vi "KeeperDefPosSkillVSS.vi"(8 "error in (no error)":errorcluster, 9 "Game":refnum<class "Game.lvclass">, 10 "Robot in":refnum<class "Robot.lvclass">, 11 "KeeperDefPosSkillVSS in":refnum<class "KeeperDefPosSkillVSS.lvclass">) -> (0 "error out":errorcluster, 2 "Robot out":refnum<class "Robot.lvclass">, 3 "KeeperDefPosSkillVSS out":refnum<class "KeeperDefPosSkillVSS.lvclass">)   [LabVIEW 2020, in "KeeperDefPosSkillVSS.lvclass"]
uses:
  KeeperDefPosSkillVSS.lvclass
  Robot_class/Robot.lvclass
  Game_class/Game.lvclass
  Utilities_class/Utilities.lvclass
  Game_class/Game.lvclass/Game.ctl
  Ball_class/Ball.lvclass/Ball.ctl
  Object_class/Object.lvclass/Object.ctl
  Robot_class/Robot.lvclass/Robot.ctl
  Game_class/Read FieldRef.vi
  Game_class/Read BallRef.vi
  Ball_class/Read v_x.vi
  Ball_class/Read v_y.vi
  Object_class/Read pos_est_y.vi
  Object_class/Read y.vi
  Object_class/Read x.vi
  Robot_class/Write dest_x.vi
  Robot_class/Write dest_y.vi
  Robot_class/Write dest_orientation.vi
  Ball_class/Ball.lvclass
  C:/Users/lucio/Desktop/Horie/ROBOIME/VSS_AI/Object_class/Object.lvclass
  Field_class/Field.lvclass
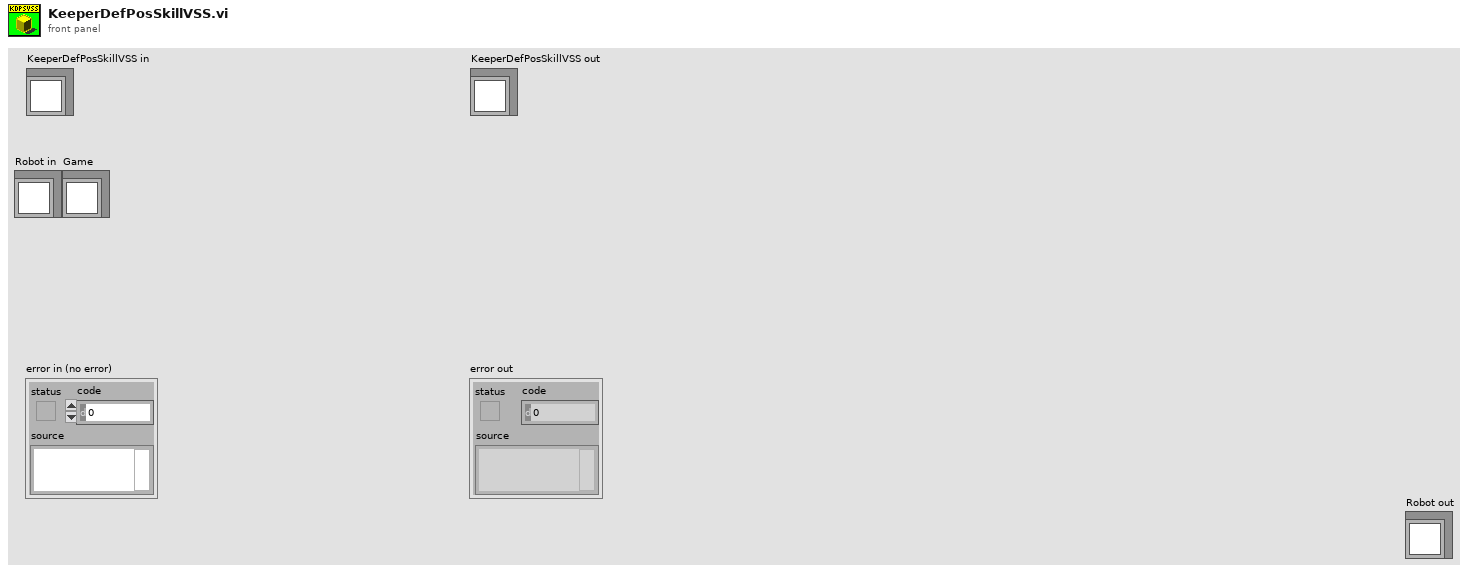
[diagram p1: front panel]
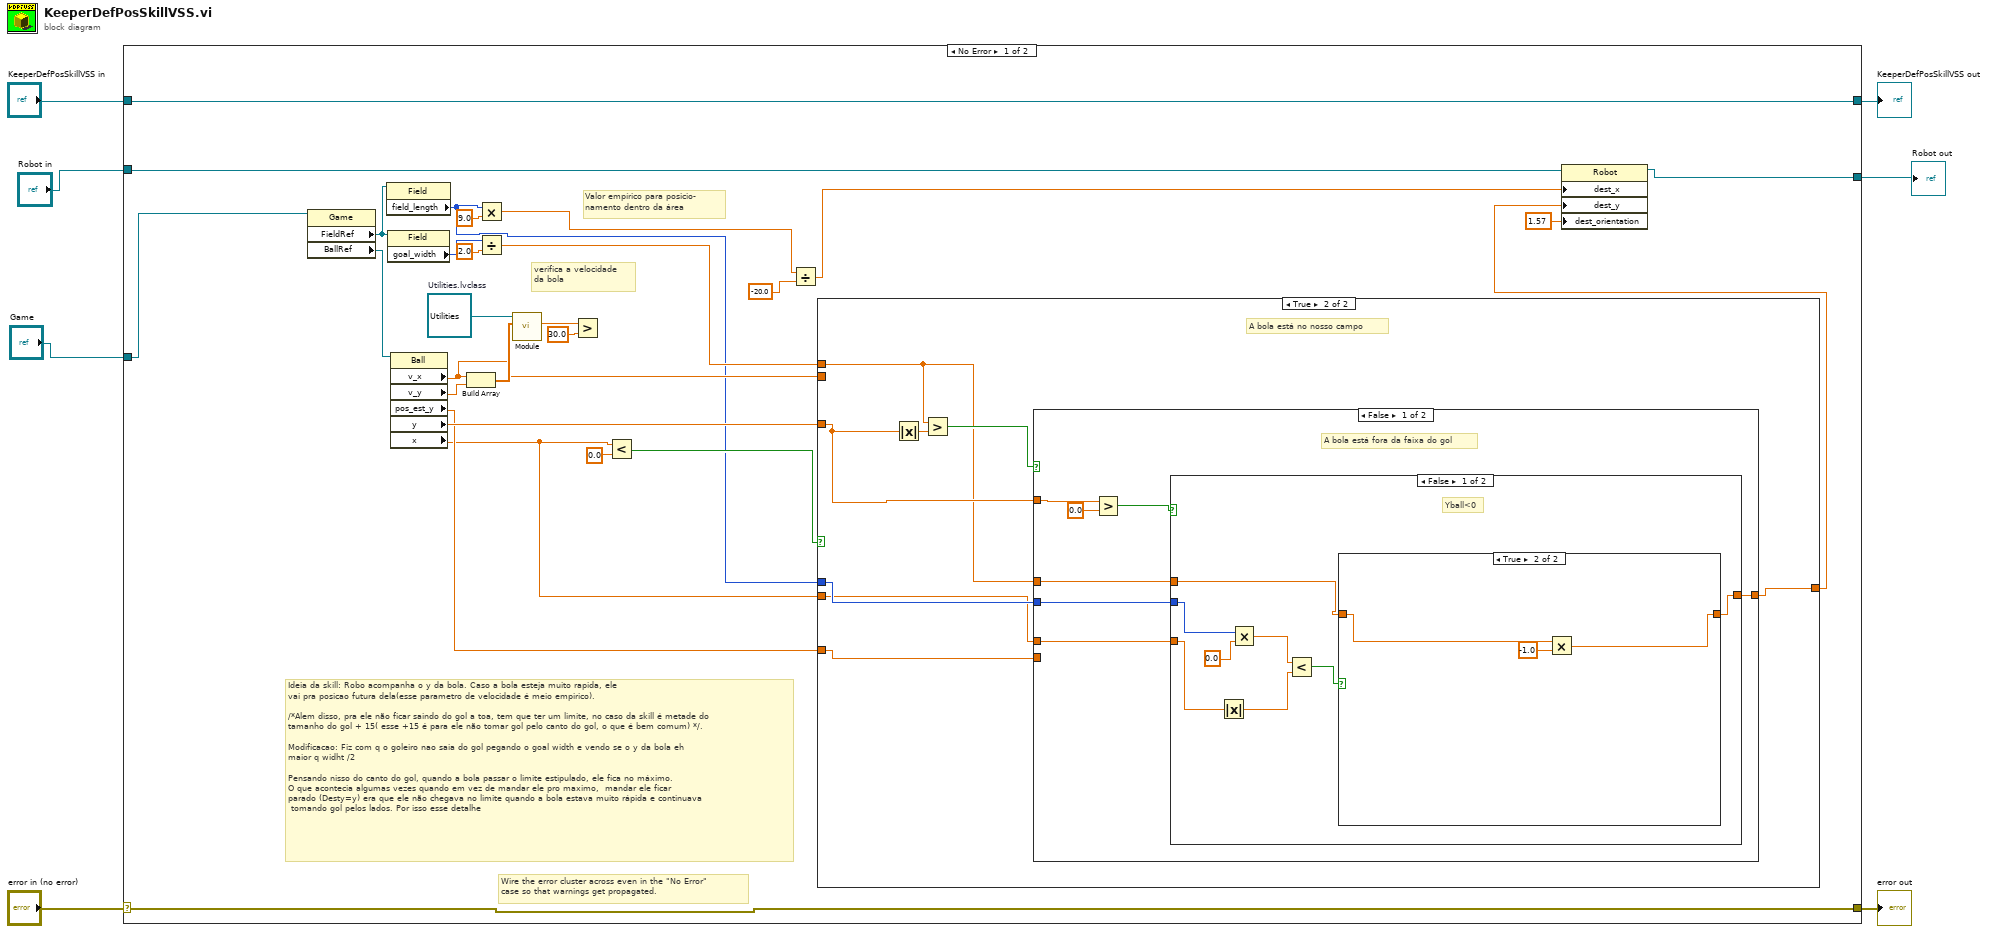
[diagram p0: block diagram]
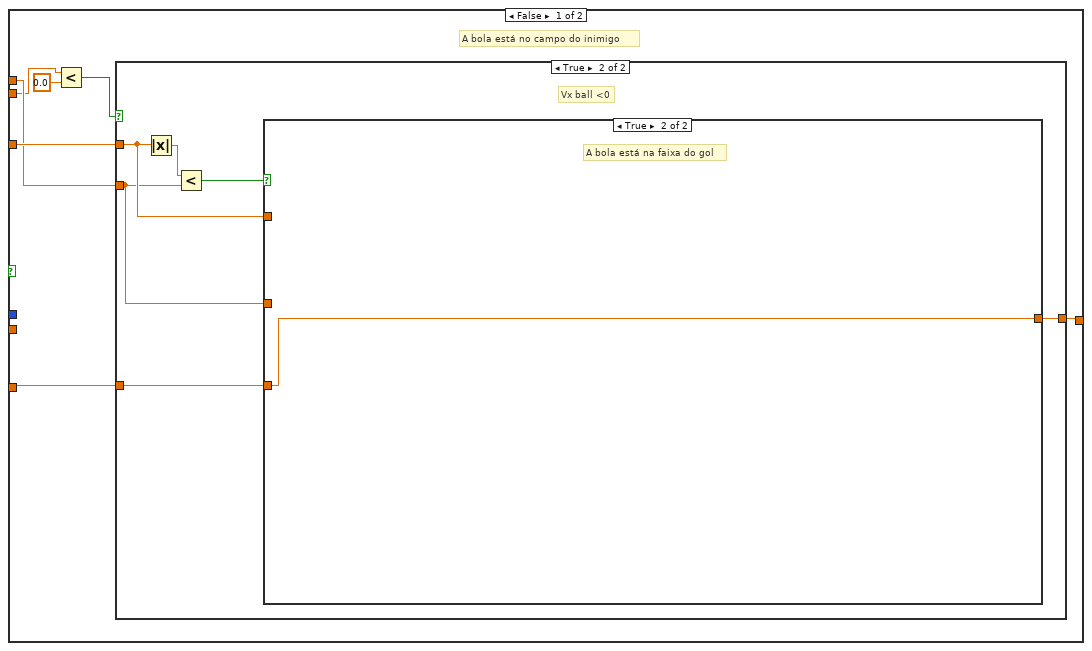
[diagram p2: hidden frame]
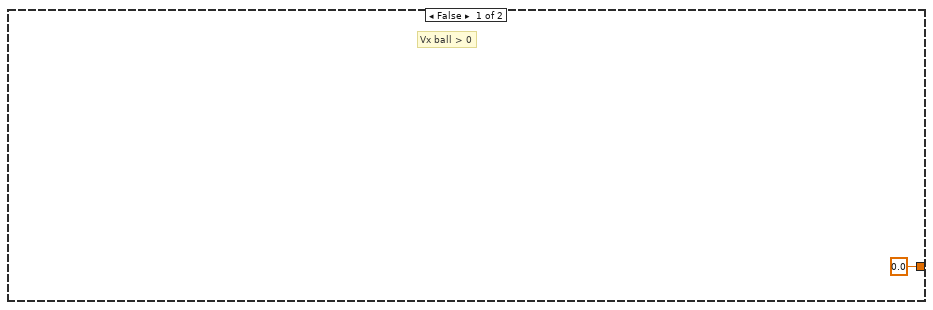
[diagram p3: hidden frame]
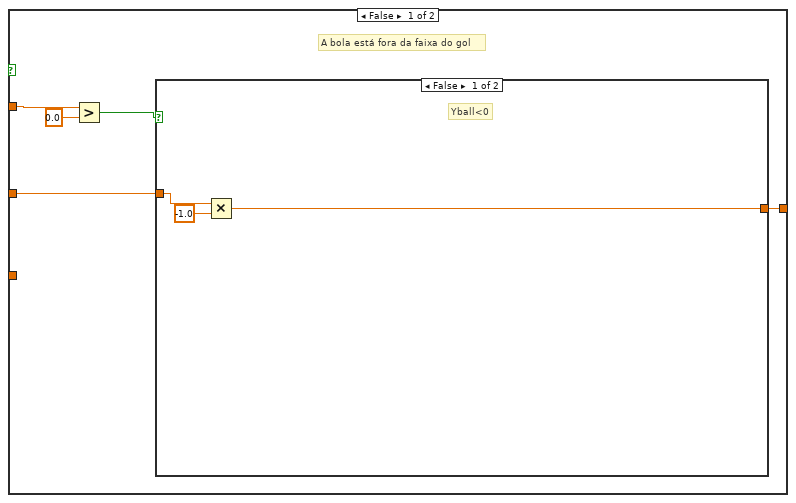
[diagram p4: hidden frame]
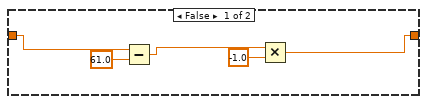
[diagram p6: hidden frame]
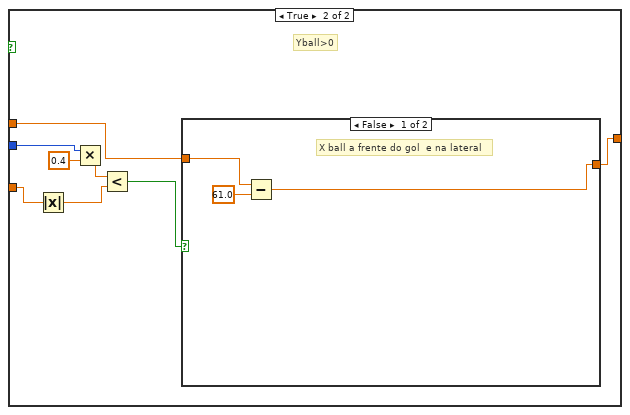
[diagram p7: hidden frame]
diagram:
  n1 = case shown="No Error" "error in (no error)" {
    selector: "error in (no error)" -> [w34 w106]
    tunnel: [w34 w106] -> w6
    tunnel: [w35 w105] -> w4
    tunnel: "KeeperDefPosSkillVSS in" -> [w35 w105]
    tunnel: "Game" -> [w27 _]
    tunnel: "Robot in" -> [w26 w104]
    tunnel: [w25 w104] -> w1
    frame No Error {
      w22 = refnum<class "Utilities.lvclass"> refnum  # Utilities.lvclass
      # "Ideia da skill: Robo acompanha o y da bola. Caso a bola esteja muito rapida, ele \nvai pra posicao futura dela(esse parametro de velocidade é meio empirico). \n\n/*Alem disso, pra ele não ficar saindo do gol a toa, tem que ter um limite, no caso da skill é metade do \ntamanho do gol + 15( esse +15 é para ele não tomar gol pelo canto do gol, o que é bem comum) */. \n\nModificacao: Fiz com q o goleiro nao saia do gol pegando o goal width e vendo se o y da bola eh \nmaior q widht /2\n\nPensando nisso do canto do gol, quando a bola passar o limite estipulado, ele fica no máximo. \nO que acontecia algumas vezes quando em vez de mandar ele pro maximo,  mandar ele ficar\nparado (Desty=y) era que ele não chegava no limite quando a bola estava muito rápida e continuava\n tomando gol pelos lados. Por isso esse detalhe"
      # "verifica a velocidade\nda bola"
      # "Valor empírico para posicio-\nnamento dentro da área"
      # "Wire the error cluster across even in the \"No Error\"\ncase so that warnings get propagated."
      n2 = property class="Game"(reference=w27) -> ("FieldRef"=w28:refnum<class "Field.lvclass">, "BallRef"=w20:refnum<class "Ball.lvclass">)  [unwired: 1 in, 2 out]
      n3 = property class="Field"(reference=w28) -> ("field_length"=w9:i32)  [unwired: 1 in, 2 out]
      n4 = property class="Field"(reference=w28) -> ("goal_width"=w24:i32)  [unwired: 1 in, 2 out]
      n5 = property class="Ball"(reference=w20) -> ("v_x"=w13:dbl, "v_y"=w19:dbl, "pos_est_y"=w10:dbl, "y"=w12:dbl, "x"=w8:dbl)  [unwired: 1 in, 2 out]
      n6 = Build Array(w13, w19) -> (w21:dbl[])
      n7 = Multiply(x=w9, y=9.0) -> (x*y=w31:dbl)
      n8 = Divide(x=w24, y=2.0) -> (x/y=w16:dbl)
      n9 = call-dynamic "Module.vi"("2D vector"=w21, "Utilities in"=w22) -> ("Modulo"=w18:dbl)  [unwired: 7 in, 2 out]
      n10 = Greater?(x=w18, y=30.0) -> ()  [unwired: 1 out]
      n11 = Less?(x=w8, y=0.0) -> (x < y?=w14:bool)
      n12 = Divide(x=w31, y=-20.0) -> (x/y=w29:dbl)
      n13 = case shown="True" w14 {
        tunnel: w16 -> [w41 w62]
        tunnel: w13 -> [w38 _]
        tunnel: w12 -> [w42 w66]
        tunnel: [w40 w63] -> w11
        tunnel: w10 -> [w39 w67]
        tunnel: w9 -> [_ w61]
        tunnel: w8 -> [_ w60]
        frame False {
          # "A bola está no campo do inimigo"
          n14 = Less?(x=w38, y=0.0 ("x")) -> (x < y?=w36:bool)
          n15 = case shown="True" w36 {
            tunnel: w42 -> [_ w47]
            tunnel: w41 -> [_ w46]
            tunnel: [0.0 ("pos_est_y") w45] -> w40
            tunnel: w39 -> [_ w44]
            frame False {
              # "Vx ball > 0"
            }
            frame True {
              # "Vx ball <0"
              n16 = Absolute Value(x=w47) -> (abs(x)=w49:dbl)
              n17 = Less?(x=w49, y=w46) -> (x < y?=w48:bool)
              n18 = case shown="True" w48 {
                tunnel: w47 -> [w54 _]
                tunnel: w46 -> [w51 _]
                tunnel: [w50 w59] -> w45
                tunnel: w44 -> [_ w59]
                frame False {
                  # "A bola está fora da faixa do gol"
                  n19 = Greater?(x=w54, y=0.0) -> (0:w52:bool)
                  n20 = case shown="False" w52 {
                    tunnel: w51 -> [w57 w58]
                    tunnel: [w55 w58] -> w50
                    frame False {
                      # "Yball<0"
                      n21 = Multiply(x=w57, y=-1.0) -> (x*y=w55:dbl)
                    }
                    frame True {
                      # "Yball>0"
                    }
                  }
                }
                frame True {
                  # "A bola está na faixa do gol"
                }
              }
            }
          }
        }
        frame True {
          # "A bola está no nosso campo"
          n22 = Absolute Value(x=w66) -> (abs(x)=w65:dbl)
          n23 = Greater?(x=w62, y=w65) -> (0:w64:bool)
          n24 = case shown="False" w64 {
            tunnel: w66 -> [w74 _]
            tunnel: w62 -> [w71 _]
            tunnel: [w70 w103] -> w63
            tunnel: w67 -> [_ w103]
            tunnel: w61 -> [w69 _]
            tunnel: w60 -> [w68 _]
            frame False {
              # "A bola está fora da faixa do gol"
              n25 = Greater?(x=w74, y=0.0) -> (0:w72:bool)
              n26 = case shown="False" w72 {
                tunnel: w71 -> [w76 w92]
                tunnel: [w75 w91] -> w70
                tunnel: w69 -> [w82 w98]
                tunnel: w68 -> [w79 w95]
                frame False {
                  # "Yball<0"
                  n27 = Absolute Value(x=w79) -> (abs(x)=w78:dbl)
                  n28 = Multiply(x=w82, y=0.0) -> (x*y=w80:dbl)
                  n29 = Less?(x=w80, y=w78) -> (x < y?=w77:bool)
                  n30 = case shown="True" w77 {
                    tunnel: w76 -> [w87 w90]
                    tunnel: [w83 w88] -> w75
                    frame False {
                      n31 = Subtract(x=w87, y=61.0) -> (x-y=w85:dbl)
                      n32 = Multiply(x=w85, y=-1.0) -> (x*y=w83:dbl)
                    }
                    frame True {
                      n33 = Multiply(x=w90, y=-1.0) -> (x*y=w88:dbl)
                    }
                  }
                }
                frame True {
                  # "Yball>0"
                  n34 = Absolute Value(x=w95) -> (abs(x)=w94:dbl)
                  n35 = Multiply(x=w98, y=0.4) -> (x*y=w96:dbl)
                  n36 = Less?(x=w96, y=w94) -> (x < y?=w93:bool)
                  n37 = case shown="False" w93 {
                    tunnel: w92 -> [w100 w102]
                    tunnel: [w99 w102] -> w91
                    frame False {
                      # "X ball a frente do gol  e na lateral"
                      n38 = Subtract(x=w100, y=61.0) -> (x-y=w99:dbl)
                    }
                    frame True {
                      # "Xball na lateral do gol"
                    }
                  }
                }
              }
            }
            frame True {
              # "A bola está na faixa do gol"
            }
          }
        }
      }
      n39 = property class="Robot"(reference=w26, "dest_x"=w29, "dest_y"=w11, "dest_orientation"=1.57) -> (reference out=w25:refnum<class "Robot.lvclass">)  [unwired: 1 in, 1 out]
    }
    frame Error {
    }
  }
  "error out" <- w6
  "KeeperDefPosSkillVSS out" <- w4
  "Robot out" <- w1
